vi "Query command.vi"(8 "error in (no error)":errorcluster, 10 "Command":string="I", 11 "VISA Refnum in":refnum<visa-resource-name>) -> (0 "error out":errorcluster, 2 "Data read":string, 3 "VISA Refnum out":refnum<visa-resource-name>)   [LabVIEW 2020, in "Arduino-Adafruit stepper.lvlib"]
uses:
  Arduino-Adafruit stepper.lvlib
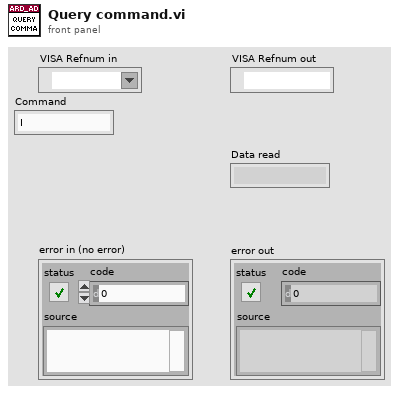
[diagram p1: front panel]
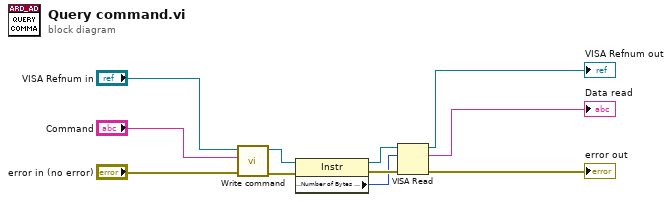
[diagram p0: block diagram]
diagram:
  n1 = call "Write command.vi"("error in"="error in (no error)", "Command"="Command", "VISA Refnum in"="VISA Refnum in") -> ("error out"=w7:errorcluster, "VISA Refnum out"=w9:refnum<visa-resource-name>)  [unwired: 6 in, 1 out]
  n2 = property class="Instr"(reference=w9, error in=w7) -> (reference out=w6:refnum<visa-resource-name>, error out=w5:errorcluster, "Serial Settings:Number of Bytes at Serial Port"=w4:u32)
  n3 = VISA Read(VISA resource name=w6, byte count=w4, error in (no error)=w5) -> (VISA resource name out=→"VISA Refnum out":refnum<visa-resource-name>, read buffer=→"Data read":string, error out=→"error out":errorcluster)  [unwired: 1 out]
